vi "Initialize Hardware References.vi"(8 "error in (no error)":errorcluster, 11 "Hardware Resources in":T1={"AIDAQ"="", "Signal Type"=enum."Sine Wave", "DODAQ"=""}) -> (0 "error out":errorcluster, 3 "Hardware Resources out":T1={"AIDAQ"="", "Signal Type"=enum."Sine Wave", "DODAQ"=""})   [LabVIEW 2023, in "Acquisition.lvlib"]
doc: "Initialize the hardware references."
uses:
  Acquisition.lvlib
  Hardware Configuration.ctl
  Signal Type.ctl
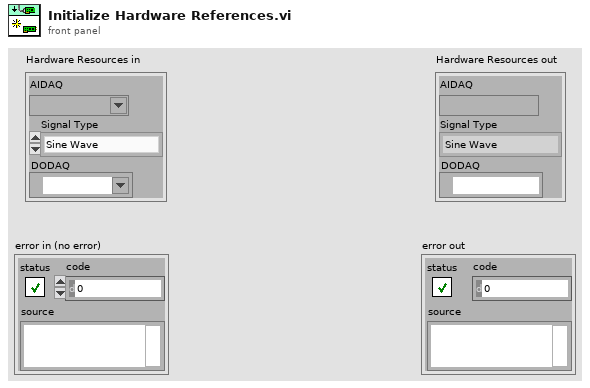
[diagram p1: front panel]
types:
  T1 = typedef "Acquisition.lvlib/Hardware Configuration.ctl" = cluster{"AIDAQ":refnum<k21>, "Signal Type":T2, "DODAQ":refnum<k21>}
  T2 = typedef "Acquisition.lvlib/Signal Type.ctl" = enum16{"cDAQ Thermistor", "cDAQ TC", "cDAQ RTD", "myDAQ Temp", "Sine Wave", "Square with Noise"}
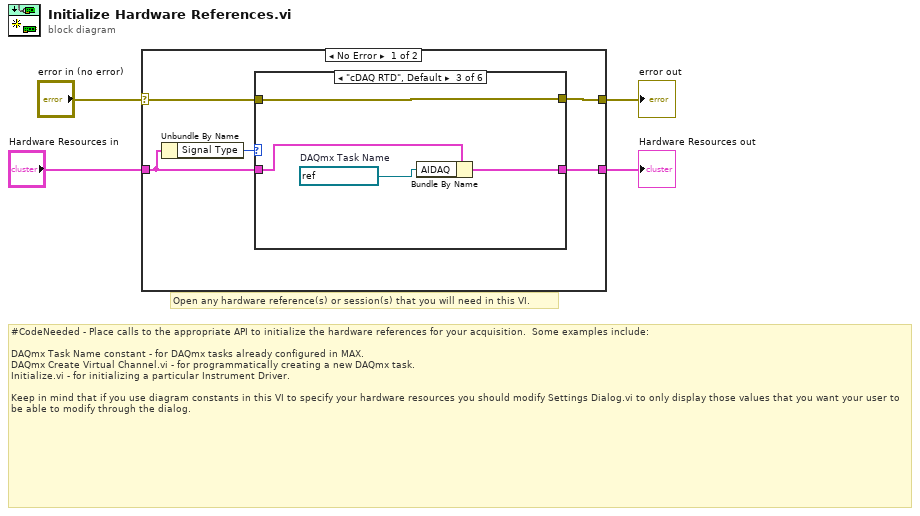
[diagram p0: block diagram]
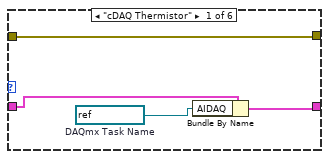
[diagram p2: hidden frame]
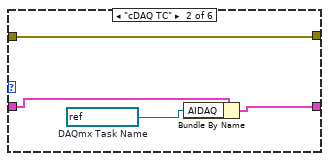
[diagram p3: hidden frame]
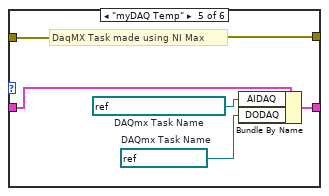
[diagram p5: hidden frame]
diagram:
  # "Open any hardware reference(s) or session(s) that you will need in this VI."
  # "#CodeNeeded - Place calls to the appropriate API to initialize the hardware references for your acquisition.  Some examples include:\n\nDAQmx Task Name constant - for DAQmx tasks already configured in MAX.\nDAQmx Create Virtual Channel.vi - for programmatically creating a new DAQmx task.\nInitialize.vi - for initializing a particular Instrument Driver.\n\nKeep in mind that if you use diagram constants in this VI to specify your hardware resources you should modify Settings Dialog.vi to only display those values that you want your user to be able to modify through the dialog."
  n1 = case shown="No Error" "error in (no error)" {
    selector: "error in (no error)" -> [w9 w31]
    tunnel: [w8 w31] -> w3
    tunnel: "Hardware Resources in" -> [w6 w32]
    tunnel: [w5 w32] -> w1
    frame No Error {
      n2 = Unbundle By Name(w6) -> ("Signal Type"=w7:T2)
      n3 = case shown="\"cDAQ RTD\", Default" w7 {
        tunnel: w9 -> [w10 w14 w18 w22 w28 w30]
        tunnel: [w10 w14 w18 w22 w28 w30] -> w8
        tunnel: w6 -> [w12 w16 w20 w23 w27 w29]
        tunnel: [w11 w15 w19 w23 w24 w29] -> w5
        frame "cDAQ Thermistor" {
          w13 = refnum<k21> "TempAI"  # DAQmx Task Name
          n4 = Bundle By Name(cluster=w12, "AIDAQ"=w13) -> (w11:T1)
        }
        frame "cDAQ TC" {
          w17 = refnum<k21> "TempTC"  # DAQmx Task Name
          n5 = Bundle By Name(cluster=w16, "AIDAQ"=w17) -> (w15:T1)
        }
        frame "cDAQ RTD", Default {
          w21 = refnum<k21> "TempRTD"  # DAQmx Task Name
          n6 = Bundle By Name(cluster=w20, "AIDAQ"=w21) -> (w19:T1)
        }
        frame "Square with Noise" {
        }
        frame "myDAQ Temp" {
          w25 = refnum<k21> "MyDAQDO"  # DAQmx Task Name
          w26 = refnum<k21> "MyDAQVoltageTask"  # DAQmx Task Name
          # "DaqMX Task made using NI Max"
          n7 = Bundle By Name(cluster=w27, "AIDAQ"=w26, "DODAQ"=w25) -> (w24:T1)
        }
        frame "Sine Wave" {
        }
      }
    }
    frame Error {
    }
  }
  "Hardware Resources out" <- w1
  "error out" <- w3
